vi "DFD Plot Group Delay.vi"(4 "group delay unit":u16(ring) items=["Samples", "Seconds"], 5 "output option":u16(ring) items=["Auto", "Floating-Point Only", "Fixed-Point Only"], 6 "fs [Hz]":dbl=-1.0 format="%.2f", 7 "# freq bins":i32=-1, 8 "error in (no error)":errorcluster, 11 "filter in":T1={"mSRate_Fs"=1.0, "mSRate_Version"="2.0", "mSRate_Comments"="", "mSRate_OrgCoef"={"type"=enum."Undefined", "gain"=1.0, "coef a (k)"=[], "coef b (v)"=[]}, "mSRate_CurCoef"={"type"=enum."Undefined", "gain"=1.0, "coef a (k)"=[], "coef b (v)"=[]}, "mSRate_Quantized?"=FALSE, "mSRate_QCoef"={"type"=enum."Undefined", "gain"=1.0, "coef a (k)"=[], "coef b (v)"=[]}, "mSRate_QSettings"=[], "mSRate_Order"=0, "mSRate_Scaling"={"mSRate_ScaleByPowerOf2?"=FALSE, "mSRate_ScaleType"=enum."No Norm"}} {"mSRate_QSettings"."source" items=["Coef a/k"=0, "Coef b/v"=7, "Input"=1, "Output"=2, "Multiplicand"=3, "Product"=4, "Sum"=5, "Delay"=6, "Gain"=8]}) -> (0 "error out":errorcluster, 2 "group delay":cluster{"f0":dbl, "df":dbl, "values":dbl[]}[](graph), 3 "filter out":T1={"mSRate_Fs"=1.0, "mSRate_Version"="2.0", "mSRate_Comments"="", "mSRate_OrgCoef"={"type"=enum."Undefined", "gain"=1.0, "coef a (k)"=[], "coef b (v)"=[]}, "mSRate_CurCoef"={"type"=enum."Undefined", "gain"=1.0, "coef a (k)"=[], "coef b (v)"=[]}, "mSRate_Quantized?"=FALSE, "mSRate_QCoef"={"type"=enum."Undefined", "gain"=1.0, "coef a (k)"=[], "coef b (v)"=[]}, "mSRate_QSettings"=[], "mSRate_Order"=0, "mSRate_Scaling"={"mSRate_ScaleByPowerOf2?"=FALSE, "mSRate_ScaleType"=enum."No Norm"}} {"mSRate_QSettings"."source" items=["Coef a/k"=0, "Coef b/v"=7, "Input"=1, "Output"=2, "Multiplicand"=3, "Product"=4, "Sum"=5, "Delay"=6, "Gain"=8]})   [LabVIEW 2017, in "NI_DigFilterLicensed.lvlib"]
doc: "Plots the group delay response of a filter."
uses:
  <vilib>/addons/Digital Filter Design/NI_DigFilterLicensed.lvlib
  <vilib>/addons/Digital Filter Design/_Objects.llb/DFD Filter Obj.ctl
  <vilib>/addons/Digital Filter Design/_Objects.llb/DFD Filter Coef.ctl
  <vilib>/addons/Digital Filter Design/_Objects.llb/DFD Filter Structure Type Selector.ctl
  <vilib>/addons/Digital Filter Design/_Objects.llb/dfd_Internal Quantization Settings.ctl
  <vilib>/addons/Digital Filter Design/_Objects.llb/dfd_Internal Quantization Srcs.ctl
  <vilib>/addons/Digital Filter Design/_Objects.llb/DFD Coef Norm Type.ctl
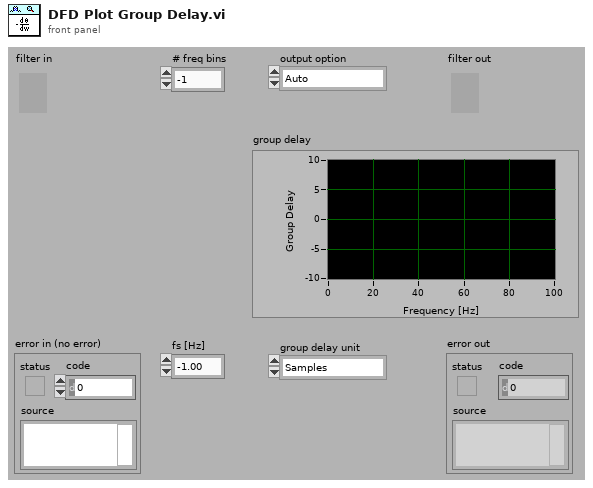
[diagram p1: front panel]
types:
  T1 = typedef "NI_DigFilterLicensed.lvlib/DFD Filter Obj.ctl" = cluster{"mSRate_Fs":dbl, "mSRate_Version":string, "mSRate_Comments":string, "mSRate_OrgCoef":T2, "mSRate_CurCoef":T2, "mSRate_Quantized?":bool, "mSRate_QCoef":T2, "mSRate_QSettings":T4[], "mSRate_Order":i32, "mSRate_Scaling":cluster{"mSRate_ScaleByPowerOf2?":bool, "mSRate_ScaleType":T6}}
  T2 = typedef "NI_DigFilterLicensed.lvlib/DFD Filter Coef.ctl" = cluster{"type":T3, "gain":dbl, "coef a (k)":dbl[], "coef b (v)":dbl[]}
  T3 = typedef "NI_DigFilterLicensed.lvlib/DFD Filter Structure Type Selector.ctl" = enum16{"Undefined", "FIR Direct Form", "FIR Direct Form Transposed", "FIR Symmetric", "FIR Antisymmetric", "IIR Direct Form I", "IIR Direct Form I Transposed", "IIR Direct Form II", "IIR Direct Form II Transposed", "IIR Cascaded Second Order Sections Form I", "IIR Cascaded Second Order Sections Form I Transposed", "IIR Cascaded Second Order Sections Form II", "IIR Cascaded Second Order Sections Form II Transposed", "Lattice Allpass (basic sections)", "Lattice Allpass (one multiplier sections)", "Lattice Allpass (normalized sections)", "Lattice AR (basic sections)", "Lattice AR (one multiplier sections)", "Lattice AR (normalized sections)", "Lattice MA (minimum phase)", "Lattice MA (maximum phase)", "Lattice ARMA (basic sections)", "Lattice ARMA (one multiplier sections)", "Lattice ARMA (normalized sections)"}
  T4 = typedef "NI_DigFilterLicensed.lvlib/dfd_Internal Quantization Settings.ctl" = cluster{"source":T5, "wl":i16, "iwl":i16, "overflow mode":enum16{"Saturation", "Wrap"}, "rounding mode":enum16{"Nearest", "Truncation"}, "signed?":bool}
  T5 = typedef "NI_DigFilterLicensed.lvlib/dfd_Internal Quantization Srcs.ctl" = u16
  T6 = typedef "NI_DigFilterLicensed.lvlib/DFD Coef Norm Type.ctl" = enum16{"No Norm", "Time Domain 1-Norm", "Time Domain 2-Norm", "Time Domain Inf-Norm"}
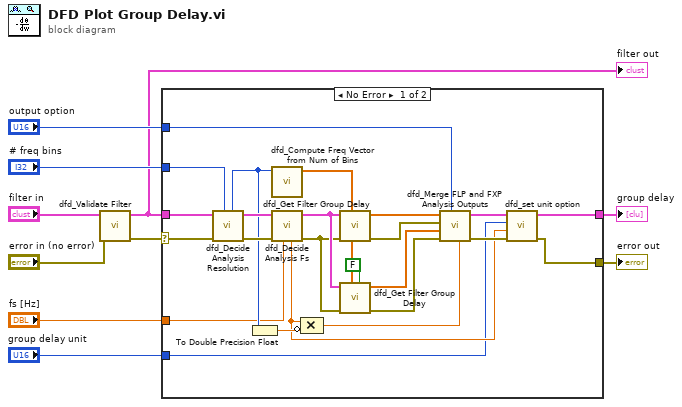
[diagram p0: block diagram]
diagram:
  n1 = call <vilib>:"dfd_Validate Filter.vi"("error in (no error)"="error in (no error)", "filter in"="filter in") -> ("error out"=w2:errorcluster, "filter out"=w4:T1)  [unwired: 1 in, 7 out]
  "filter out" <- w4
  n2 = case shown="No Error" w2 {
    selector: w2 -> [w32 w35]
    tunnel: w4 -> [w33 _]
    tunnel: "fs [Hz]" -> [w19 _]
    tunnel: "# freq bins" -> [w30 _]
    tunnel: "output option" -> [w25 _]
    tunnel: [w13 _] -> w7
    tunnel: [w15 w35] -> w6
    tunnel: "group delay unit" -> [w11 _]
    frame No Error {
      n3 = call <vilib>:"dfd_Decide Analysis Resolution.vi"("# freq bins in"=w30, "error in (no error)"=w32, "filter in"=w33) -> ("error out"=w31:errorcluster, "filter out"=w34:T1, "# freq bins out"=w21:i32)  [unwired: 3 in, 3 out]
      n4 = To Double Precision Float(number=w21) -> (double precision float=w18:dbl)
      n5 = call <vilib>:"dfd_Compute Freq Vector from Num of Bins.vi"("# freq bins (512)"=w21) -> ("freq points"=w17:dbl[])  [unwired: 10 out]
      n6 = call <vilib>:"dfd_Decide Analysis Fs.vi"("fs in [Hz]"=w19, "error in (no error)"=w31, "filter in"=w34) -> ("error out"=w27:errorcluster, "filter out"=w28:T1, "fs out [Hz]"=w12:dbl)  [unwired: 1 in, 5 out]
      n7 = Compound Arithmetic op=MULTIPLY(w12, invert w18) -> (w20:dbl)
      n8 = call <vilib>:"dfd_Get Filter Group Delay.vi"("freq points [Hz]"=w17, "error in (no error)"=w27, "filter in"=w28) -> ("error out"=w24:errorcluster, "group delay"=w26:dbl[])  [unwired: 2 in, 5 out]
      n9 = call <vilib>:"dfd_Get Filter Group Delay.vi"("output option\n(T: FLP)"=FALSE ("output option\n(T: FLP)"), "freq points [Hz]"=w17, "error in (no error)"=w27, "filter in"=w28) -> ("error out"=w22:errorcluster, "group delay"=w23:dbl[])  [unwired: 1 in, 5 out]
      n10 = call <vilib>:"dfd_Merge FLP and FXP Analysis Outputs.vi"("delta"=w20, "output option"=w25, "error in FXP"=w22, "response FXP"=w23, "error in FLP"=w24, "response FLP"=w26) -> ("error out"=w16:errorcluster, "freq responses"=w14:cluster{"f0":dbl, "df":dbl, "values":dbl[]}[])  [unwired: 4 out]
      n11 = call <vilib>:"dfd_set unit option.vi"("error in (no error)"=w16, "fs [Hz]"=w12, "unit option"=w11, "freq responses"=w14) -> ("error out"=w15:errorcluster, "freq responses out"=w13:cluster{"f0":dbl, "df":dbl, "values":dbl[]}[])  [unwired: 6 out]
    }
    frame Error {
    }
  }
  "error out" <- w6
  "group delay" <- w7
